vi "INIT Parse Test Config.vi"(8 "error in (no error)":errorcluster, 9 "Pump CtlRef In":T3, 10 "All XL Input":string[][](array[string])=[["TEST#", "OLR001", "A Fill Lo", "A Fill Hi", "A Resist", "A Tolerence", "A Drain Lo", "A Drain Hi", "A Resist", "A Tolerence", "B Fill Lo", "B Fill Hi", "B Resist", "B  Tolerence", "B Drain Lo", "B Drain Hi", "B Resist", "B Tolerence", "", ""], ["Step Levels", "0.78", "7.910", "8.010", "100", "2", "7.550", "7.650", "100", "2", "7.685", "7.785", "100", "2", "2", "7.425", "100", "2", "", ""], ["Tolerence", "0.01", "7.460", "7.560", "200", "3", "7.100", "7.200", "200", "3", "7.235", "7.335", "200", "3", "3", "6.975", "200", "3", "", ""], ["Sample Rate", "0.1", "7.010", "7.110", "300", "4", "6.650", "6.750", "300", "4", "6.785", "6.885", "300", "4", "4", "6.525", "300", "4", "", ""], ["Resistor", "100", "6.560", "6.660", "400", "5", "6.200", "6.300", "400", "5", "6.335", "6.435", "400", "5", "5", "6.075", "400", "5", "", ""], ["M Level cal", "1", "6.110", "6.210", "500", "6", "5.750", "5.850", "500", "6", "5.885", "5.985", "500", "6", "6", "5.625", "500", "6", "", ""], ["B Level cal", "0", "5.660", "5.760", "600", "7", "5.300", "5.400", "600", "7", "5.435", "5.535", "600", "7", "7", "5.175", "600", "7", "", ""], ["Max Fill Rate", "0.1", "5.210", "5.310", "700", "8", "4.850", "4.950", "700", "8", "4.985", "5.085", "700", "8", "8", "4.725", "700", "8", "", ""], ["Max Gal", "10", "4.760", "4.860", "800", "9", "4.400", "4.500", "800", "9", "4.535", "4.635", "800", "9", "9", "4.275", "800", "9", "", ""], ["Max Inches", "10", "4.310", "4.410", "900", "10", "3.950", "4.050", "900", "10", "4.085", "4.185", "900", "10", "10", "3.825", "900", "10", "", ""], ["Rows", "12", "3.860", "3.960", "1000", "11", "3.500", "3.600", "1000", "11", "3.635", "3.735", "1000", "11", "11", "3.375", "1000", "11", "", ""], ["Cols", "18", "3.410", "3.510", "1100", "12", "3.050", "3.150", "1100", "12", "3.185", "3.285", "1100", "12", "12", "2.925", "1100", "12", "", ""], ["", "", "", "", "", "", "", "", "", "", "", "", "", "", "", "", "", "", "", ""], ["", "", "", "", "", "", "", "", "", "", "", "", "", "", "", "", "", "", "", ""], ["", "", "", "", "", "", "", "", "", "", "", "", "", "", "", "", "", "", "", ""], ["", "", "", "", "", "", "", "", "", "", "", "", "", "", "", "", "", "", "", ""], ["", "", "", "", "", "", "", "", "", "", "", "", "", "", "", "", "", "", "", ""], ["", "", "", "", "", "", "", "", "", "", "", "", "", "", "", "", "", "", "", ""], ["", "", "", "", "", "", "", "", "", "", "", "", "", "", "", "", "", "", "", ""], ["", "", "", "", "", "", "", "", "", "", "", "", "", "", "", "", "", "", "", ""], ["", "", "", "", "", "", "", "", "", "", "", "", "", "", "", "", "", "", "", ""], ["", "", "", "", "", "", "", "", "", "", "", "", "", "", "", "", "", "", "", ""], ["", "", "", "", "", "", "", "", "", "", "", "", "", "", "", "", "", "", "", ""], ["", "", "", "", "", "", "", "", "", "", "", "", "", "", "", "", "", "", "", ""], ["", "", "", "", "", "", "", "", "", "", "", "", "", "", "", "", "", "", "", ""], ["", "", "", "", "", "", "", "", "", "", "", "", "", "", "", "", "", "", "", ""], ["", "", "", "", "", "", "", "", "", "", "", "", "", "", "", "", "", "", "", ""], ["", "", "", "", "", "", "", "", "", "", "", "", "", "", "", "", "", "", "", ""]], 11 "Bench Status":T4) -> (0 "error out":errorcluster, 2 "Full Config":T2)   [LabVIEW 2024]
uses:
  Control Definitions/Def PumpCtlRefs.ctl
  Control Definitions/Def Bench Status.ctl
  Control Definitions/Def BenchCfg.ctl
  Control Definitions/Def FullCfg.ctl
panel:
  in  "Bench Config":T1
  out "Bench Config":T1
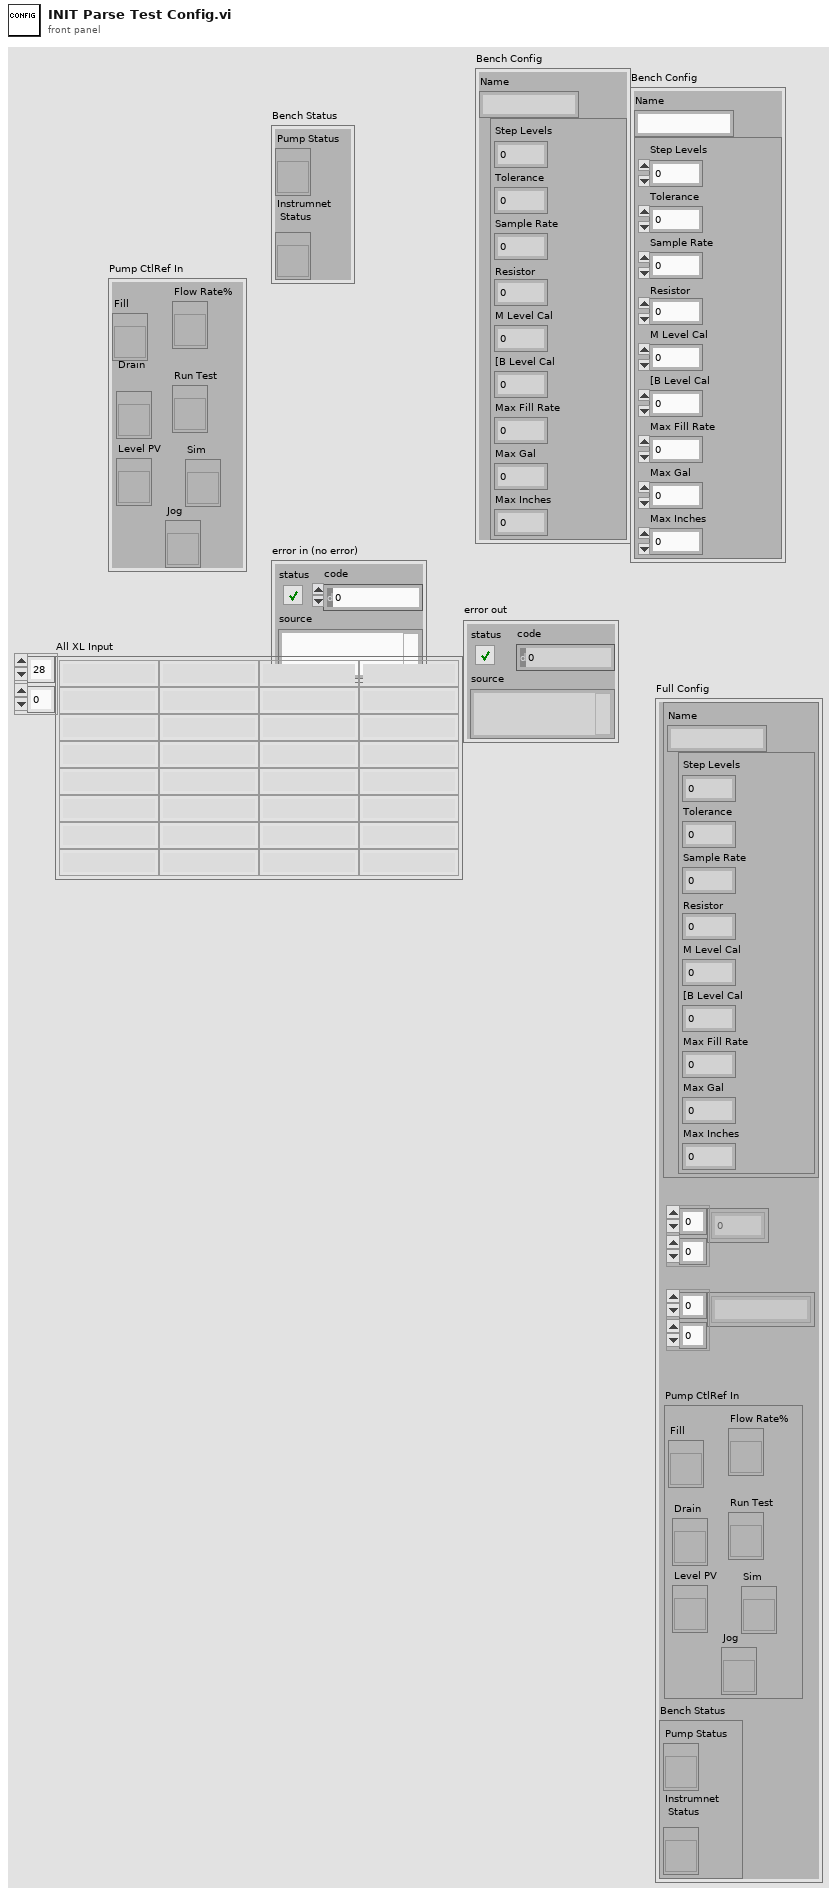
[diagram p1: front panel]
types:
  T1 = typedef "Def BenchCfg.ctl" = cluster{"Name":string, cluster{"Step Levels":dbl, "Tolerance":dbl, "Sample Rate":dbl, "Resistor":dbl, "M Level Cal":dbl, "[B Level Cal":dbl, "Max Fill Rate":dbl, "Max Gal":dbl, "Max Inches":dbl}}
  T2 = typedef "Def FullCfg.ctl" = cluster{"Bench Config":T1, "Test Value Table ":dbl[][], "Table Col Titles":string[][], "Pump CtlRef In":T3, "Bench Status":T4}
  T3 = typedef "Def PumpCtlRefs.ctl" = cluster{"Fill ":refnum<vi>, "Drain":refnum<vi>, "Level PV":refnum<vi>, "Flow Rate%":refnum<vi>, "Run Test":refnum<vi>, "Sim":refnum<vi>, "Jog":refnum<vi>}
  T4 = typedef "Def Bench Status.ctl" = cluster{"Pump Status":refnum<vi>, "Instrumnet\n Status":refnum<vi>}
  T5 = cluster{"String":string, cluster{"[0]":dbl, "[1]":dbl, "[2]":dbl, "[3]":dbl, "[4]":dbl, "[5]":dbl, "[6]":dbl, "[7]":dbl, "[8]":dbl}}
  T6 = cluster{"[0]":dbl, "[1]":dbl, "[2]":dbl, "[3]":dbl, "[4]":dbl, "[5]":dbl, "[6]":dbl, "[7]":dbl, "[8]":dbl}
  T7 = cluster{"Bench Config":T1, dbl[][], string[][], "Pump CtlRef In":T3, "Bench Status":T4}
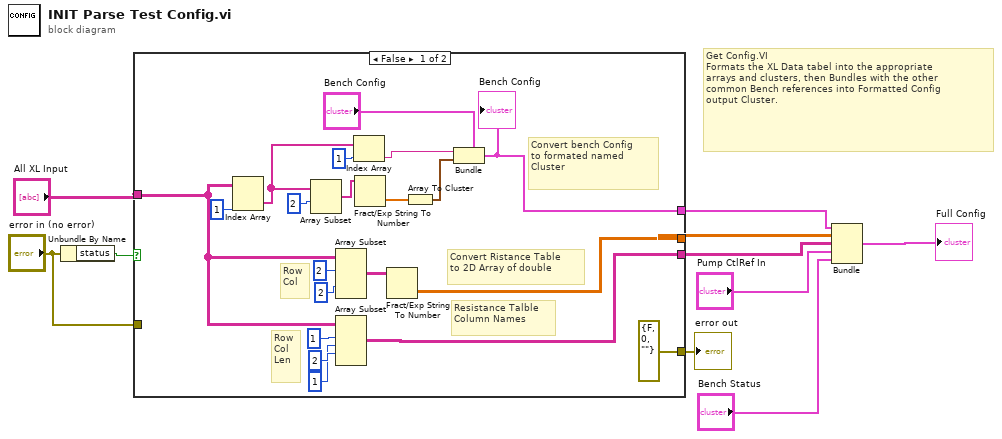
[diagram p0: block diagram]
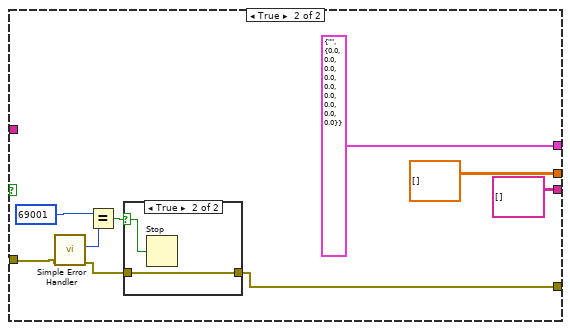
[diagram p2: hidden frame]
diagram:
  # "Get Config.VI\nFormats the XL Data tabel into the appropriate\narrays and clusters, then Bundles with the other\ncommon Bench references into Formatted Config\noutput Cluster."
  n1 = Unbundle By Name("error in (no error)") -> ("status"=w10:bool)
  n2 = case shown="False" w10 {
    tunnel: "All XL Input" -> [w19 _]
    tunnel: [w25 dbl[][] []] -> w7
    tunnel: [w15 T5 {"String"="", {"[0]"=0.0, "[1]"=0.0, "[2]"=0.0, "[3]"=0.0, "[4]"=0.0, "[5]"=0.0, "[6]"=0.0, "[7]"=0.0, "[8]"=0.0}}] -> w3
    tunnel: "error in (no error)" -> [_ w36]
    tunnel: [errorcluster {"status"=FALSE, "code"=0, "source"=""} ("error out") w33] -> w8
    tunnel: [w20 string[][] []] -> w4
    frame False {
      # "Resistance Talble\nColumn Names"
      # "Convert bench Config\nto formated named\nCluster"
      # "Convert Ristance Table\nto 2D Array of double"
      # "Row\nCol\nLen"
      # "Row\nCol"
      n3 = Index Array(array=w19, index (col)=1 ("index (page)")) -> (element=w14:string[])  [unwired: 1 in]
      n4 = Array Subset(array=w14, index=2) -> (w12:string[])  [unwired: 1 in]
      n5 = Array Subset(array=w19, index (row)=2 ("index"), index (col)=2 ("index")) -> (w24:string[][])  [unwired: 2 in]
      n6 = Array Subset(array=w19, index (row)=1 ("index"), length (row)=1 ("index"), index (col)=2 ("index")) -> (w20:string[][])  [unwired: 1 in]
      n7 = Index Array(array=w14, index=1) -> (element=w16:string)
      n8 = Fract/Exp String To Number(string=w12) -> (number=w28:dbl[])  [unwired: 3 in, 1 out]
      n9 = Fract/Exp String To Number(string=w24) -> (number=w25:dbl[][])  [unwired: 3 in, 1 out]
      n10 = Array To Cluster(array=w28) -> (cluster=w17:T6)
      n11 = Bundle(cluster="Bench Config", "Name"=w16, w17) -> (w15:T1)
      "Bench Config" <- w15
    }
    frame True {
      n12 = call <vilib>:"Simple Error Handler.vi"("error in (no error)"=w36) -> ("code out"=w35:i32, "error out"=w34:errorcluster)  [unwired: 4 in, 3 out]
      n13 = Equal?(x=69001 ("code"), y=w35) -> (x = y?=w37:bool)
      n14 = case shown="True" w37 {
        selector: w37 -> [_ w42]
        tunnel: w34 -> [w40 w41]
        tunnel: [w40 w41] -> w33
        frame False {
        }
        frame True {
          n15 = Stop(stop? (T)=w42) -> ()
        }
      }
    }
  }
  "error out" <- w8
  n16 = Bundle("Bench Config"=w3, w7, w4, "Pump CtlRef In"="Pump CtlRef In", "Bench Status"="Bench Status") -> (→"Full Config":T7)  [unwired: 1 in]
